vi "subVI_CONEX_getLimits.vi"(0 "CONEX Cluster":T1, 3 "Error IN":errorcluster) -> (4 "Retract Limit":dbl[](array[numeric]), 6 "CONEX Cluster out":T1, 8 "Extend Limit":dbl[](array[numeric]), 9 "error out":errorcluster)   [LabVIEW 2010]
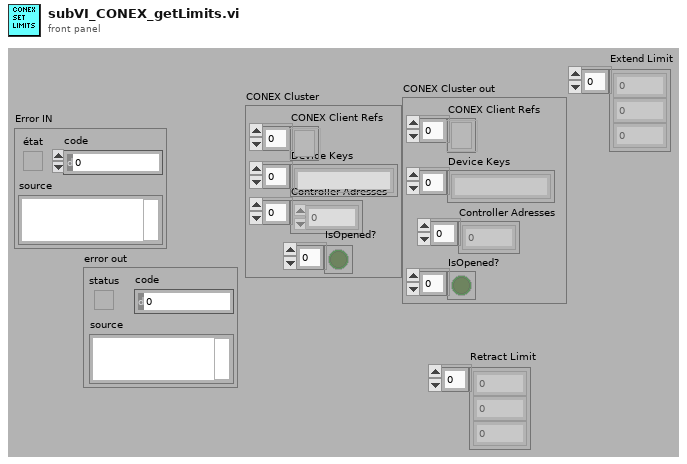
[diagram p1: front panel]
types:
  T1 = cluster{"CONEX Client Refs":refnum<k24>[], "Device Keys":string[], "Controller Adresses":i32[], "IsOpened?":bool[]}
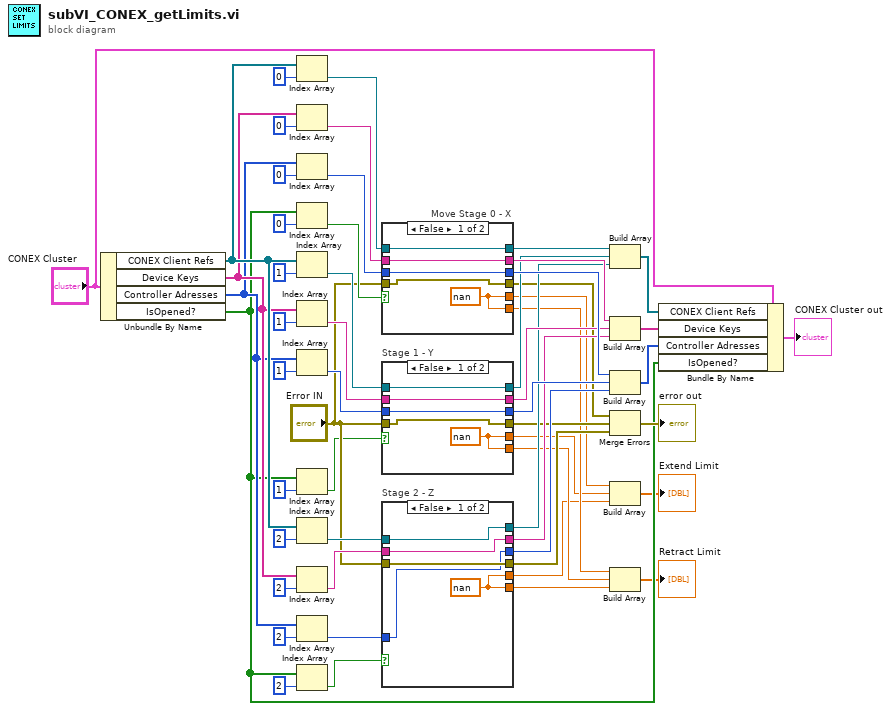
[diagram p0: block diagram]
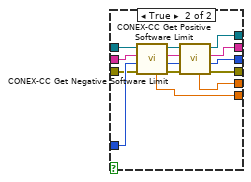
[diagram p2: hidden frame]
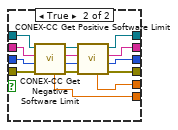
[diagram p3: hidden frame]
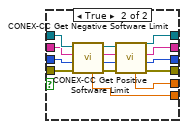
[diagram p4: hidden frame]
diagram:
  n1 = Unbundle By Name("CONEX Cluster") -> ("CONEX Client Refs"=w52:refnum<k24>[], "Device Keys"=w47:string[], "Controller Adresses"=w42:i32[], "IsOpened?"=w11:bool[])
  n2 = Index Array(array=w52, index=0) -> (element=w51:refnum<k24>)
  n3 = Index Array(array=w47, index=0) -> (element=w46:string)
  n4 = Index Array(array=w42, index=0) -> (element=w41:i32)
  n5 = Index Array(array=w11, index=0) -> (element=w32:bool)
  n6 = Index Array(array=w52, index=1) -> (element=w30:refnum<k24>)
  n7 = Index Array(array=w47, index=1) -> (element=w28:string)
  n8 = Index Array(array=w42, index=1) -> (element=w25:i32)
  n9 = Index Array(array=w11, index=1) -> (element=w9:bool)
  n10 = Index Array(array=w52, index=2) -> (element=w29:refnum<k24>)
  n11 = Index Array(array=w47, index=2) -> (element=w27:string)
  n12 = Index Array(array=w42, index=2) -> (element=w26:i32)
  n13 = Index Array(array=w11, index=2) -> (element=w12:bool)
  n14 = case "Move Stage 0 - X" shown="False" w32 {
    tunnel: w51 -> [w57 w74]
    tunnel: w46 -> [w58 w73]
    tunnel: w41 -> [w59 w72]
    tunnel: "Error IN" -> [w60 w71]
    tunnel: [w57 w66] -> w40
    tunnel: [w58 w65] -> w39
    tunnel: [w59 w64] -> w38
    tunnel: [w60 w63] -> w14
    tunnel: [w56 w62] -> w8
    tunnel: [w56 w61] -> w2
    frame False {
      w56 = nan ("Current position")
    }
    frame True {
      n15 = call <userlib>:"CONEX-CC Get Negative Software Limit.vi"("CONEX Client Ref IN"=w74, "deviceKey IN"=w73, "Address IN"=w72, "Error IN"=w71) -> ("Left limit"=w62:dbl, "CONEX Client Ref OUT"=w70:refnum<k24>, "deviceKey OUT"=w69:string, "Address OUT"=w68:i32, "Error OUT"=w67:errorcluster)  [unwired: 1 in]
      n16 = call <userlib>:"CONEX-CC Get Positive Software Limit.vi"("CONEX Client Ref IN"=w70, "deviceKey IN"=w69, "Address IN"=w68, "Error IN"=w67) -> ("Right limit"=w61:dbl, "CONEX Client Ref OUT"=w66:refnum<k24>, "deviceKey OUT"=w65:string, "Address OUT"=w64:i32, "Error OUT"=w63:errorcluster)  [unwired: 1 in]
    }
  }
  n17 = case "Stage 1 - Y" shown="False" w9 {
    tunnel: w30 -> [w76 w93]
    tunnel: w28 -> [w77 w92]
    tunnel: w25 -> [w78 w91]
    tunnel: "Error IN" -> [w79 w90]
    tunnel: [w76 w85] -> w18
    tunnel: [w77 w84] -> w21
    tunnel: [w78 w83] -> w22
    tunnel: [w79 w82] -> w17
    tunnel: [w75 w81] -> w7
    tunnel: [w75 w80] -> w3
    frame False {
      w75 = nan ("Current position")
    }
    frame True {
      n18 = call <userlib>:"CONEX-CC Get Negative Software Limit.vi"("CONEX Client Ref IN"=w93, "deviceKey IN"=w92, "Address IN"=w91, "Error IN"=w90) -> ("Left limit"=w81:dbl, "CONEX Client Ref OUT"=w86:refnum<k24>, "deviceKey OUT"=w87:string, "Address OUT"=w88:i32, "Error OUT"=w89:errorcluster)  [unwired: 1 in]
      n19 = call <userlib>:"CONEX-CC Get Positive Software Limit.vi"("CONEX Client Ref IN"=w86, "deviceKey IN"=w87, "Address IN"=w88, "Error IN"=w89) -> ("Right limit"=w80:dbl, "CONEX Client Ref OUT"=w85:refnum<k24>, "deviceKey OUT"=w84:string, "Address OUT"=w83:i32, "Error OUT"=w82:errorcluster)  [unwired: 1 in]
    }
  }
  n20 = case "Stage 2 - Z" shown="False" w12 {
    tunnel: w29 -> [w95 w112]
    tunnel: w27 -> [w96 w111]
    tunnel: w26 -> [w97 w110]
    tunnel: "Error IN" -> [w98 w109]
    tunnel: [w95 w104] -> w19
    tunnel: [w96 w103] -> w20
    tunnel: [w97 w102] -> w23
    tunnel: [w98 w101] -> w16
    tunnel: [w94 w100] -> w6
    tunnel: [w94 w99] -> w4
    frame False {
      w94 = nan ("Current position")
    }
    frame True {
      n21 = call <userlib>:"CONEX-CC Get Negative Software Limit.vi"("CONEX Client Ref IN"=w112, "deviceKey IN"=w111, "Address IN"=w110, "Error IN"=w109) -> ("Left limit"=w100:dbl, "CONEX Client Ref OUT"=w105:refnum<k24>, "deviceKey OUT"=w106:string, "Address OUT"=w108:i32, "Error OUT"=w107:errorcluster)  [unwired: 1 in]
      n22 = call <userlib>:"CONEX-CC Get Positive Software Limit.vi"("CONEX Client Ref IN"=w105, "deviceKey IN"=w106, "Address IN"=w108, "Error IN"=w107) -> ("Right limit"=w99:dbl, "CONEX Client Ref OUT"=w104:refnum<k24>, "deviceKey OUT"=w103:string, "Address OUT"=w102:i32, "Error OUT"=w101:errorcluster)  [unwired: 1 in]
    }
  }
  n23 = Build Array(w40, w18, w19) -> (w37:refnum<k24>[])
  n24 = Build Array(w39, w21, w20) -> (w36:string[])
  n25 = Build Array(w38, w22, w23) -> (w35:i32[])
  n26 = Merge Errors(w14, w17, w16) -> (→"error out":errorcluster)
  n27 = Build Array(w2, w3, w4) -> (→"Extend Limit":dbl[])
  n28 = Build Array(w8, w7, w6) -> (→"Retract Limit":dbl[])
  n29 = Bundle By Name(cluster="CONEX Cluster", "CONEX Client Refs"=w37, "Device Keys"=w36, "Controller Adresses"=w35, "IsOpened?"=w11) -> (→"CONEX Cluster out":T1)
